vi "TreeControl.vi"() -> ()   [LabVIEW 2018]
panel:
  in  "Tree":string(tree)
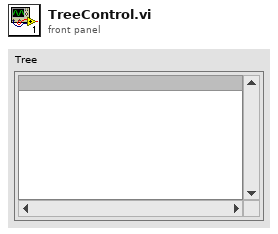
[diagram p1: front panel]
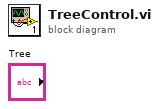
[diagram p0: block diagram]
diagram:
